vi "Get XNET Signal Names.vi"(6 "Add Info?":bool, 7 "Parent Ref in":T1 format="%.0x", 8 "error in":errorcluster, 9 "Tree In":refnum<vi>, 10 "Parent":string, 11 "Frms":refnum<k21>[](array[refnum])) -> (0 "error out":errorcluster, 1 "Tree Out":refnum<vi>, 3 "XNET Signal Names":refnum<k21>[](array[refnum]))   [LabVIEW 2015, in "Protection and Rolling Counter Addon System Explorer.lvlib"]
uses:
  Protection and Rolling Counter Addon System Explorer.lvlib
  <vilib>/NI Veristand/Custom Device API/Custom Device Item Ref.ctl
  <vilib>/NI Veristand/Custom Device API/Custom Device Channel.ctl
  <vilib>/NI Veristand/Custom Device API/Custom Device Channel Type.ctl
  Shared/SubVIs/GUID Lookup.vi
  <vilib>/NI Veristand/Custom Device API/Set Item Property (U32).vi
  <resource>/objmgr/xnet.rc
  <vilib>/NI Veristand/Custom Device API/Custom Device API.lvlib
  Shared/Protection and Rolling Counter Addon Shared.lvlib
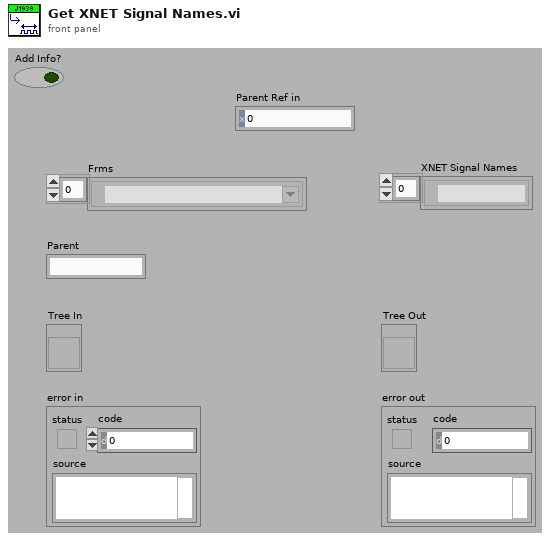
[diagram p1: front panel]
types:
  T1 = typedef "Custom Device API.lvlib/Custom Device Item Ref.ctl" = u64
  T2 = typedef "Custom Device API.lvlib/Custom Device Channel.ctl" = cluster{"Type":T3, "Units":string, "Default Value":dbl, "Faultable":bool, "Scalable":bool}
  T3 = typedef "Custom Device API.lvlib/Custom Device Channel Type.ctl" = enum16{"Input", "Output"}
  T4 = typedef "Custom Device API.lvlib/Custom Device Item Info.ctl" = cluster{"Name":string, "Is Channel":bool, "GUID":string, "Is Waveform":bool}
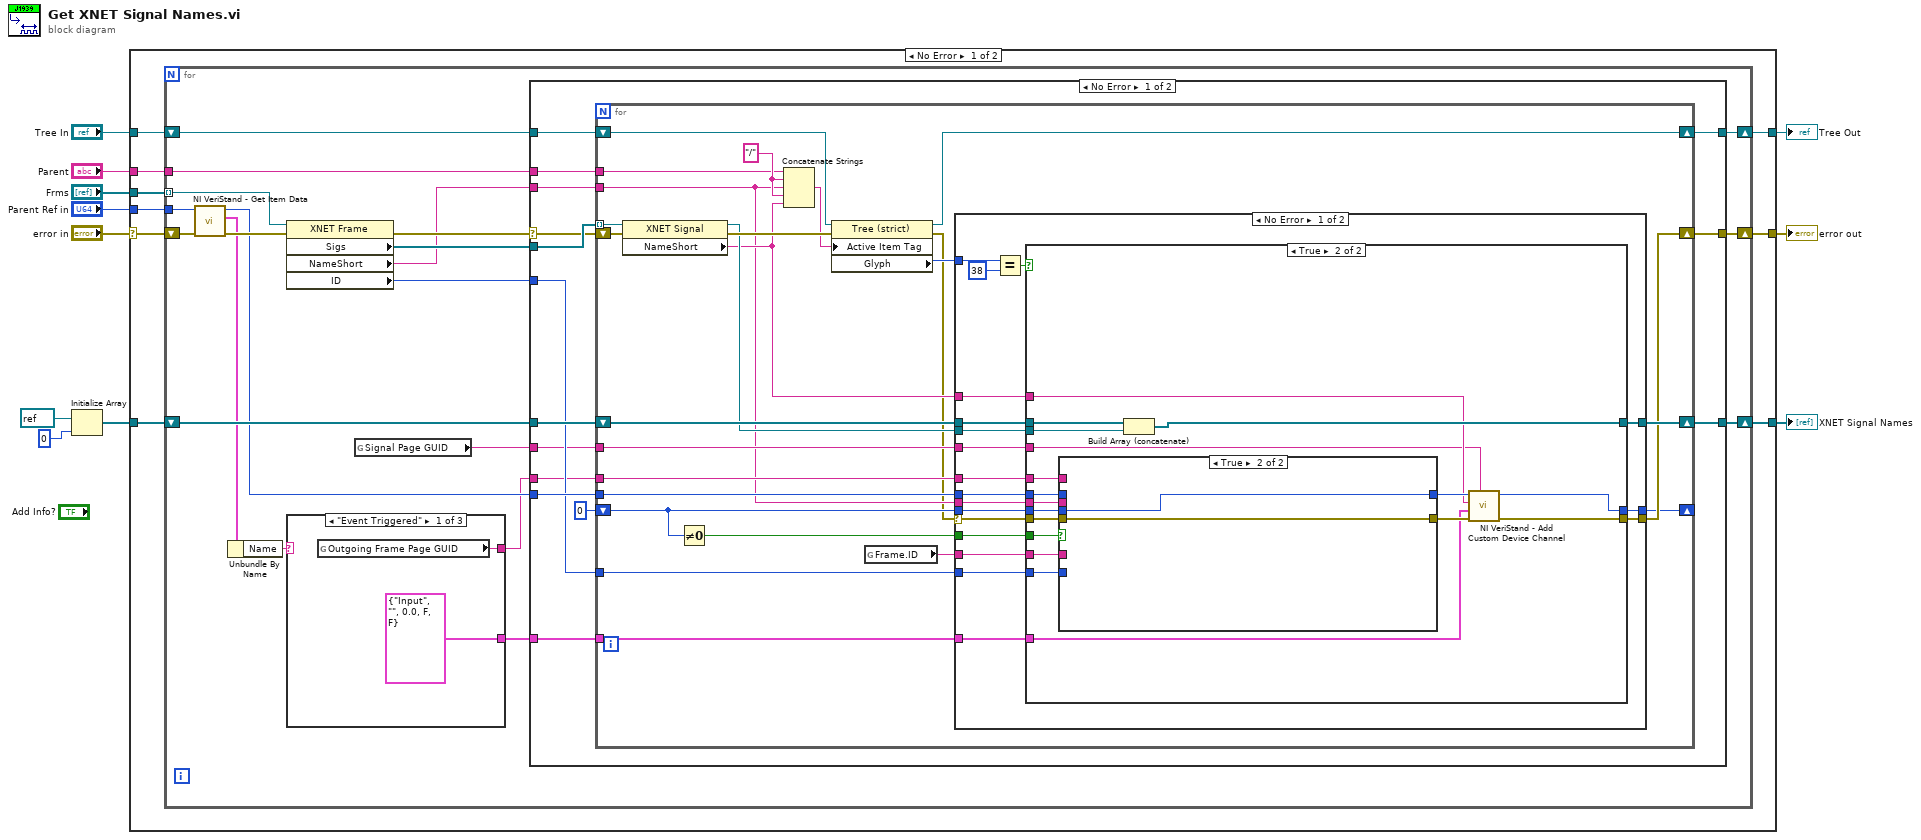
[diagram p0: block diagram]
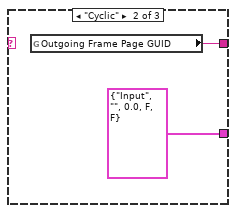
[diagram p2: hidden frame]
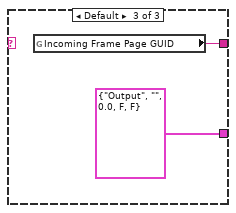
[diagram p3: hidden frame]
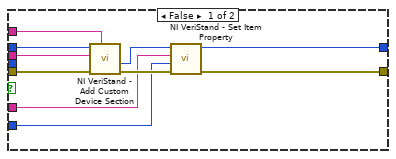
[diagram p5: hidden frame]
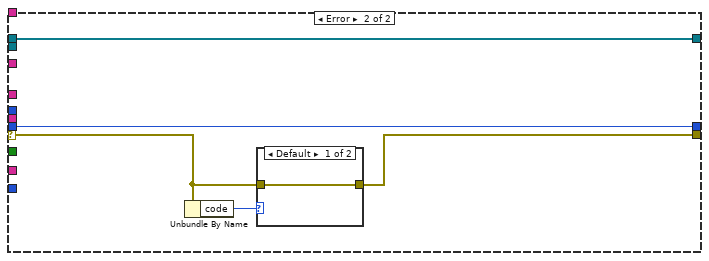
[diagram p6: hidden frame]
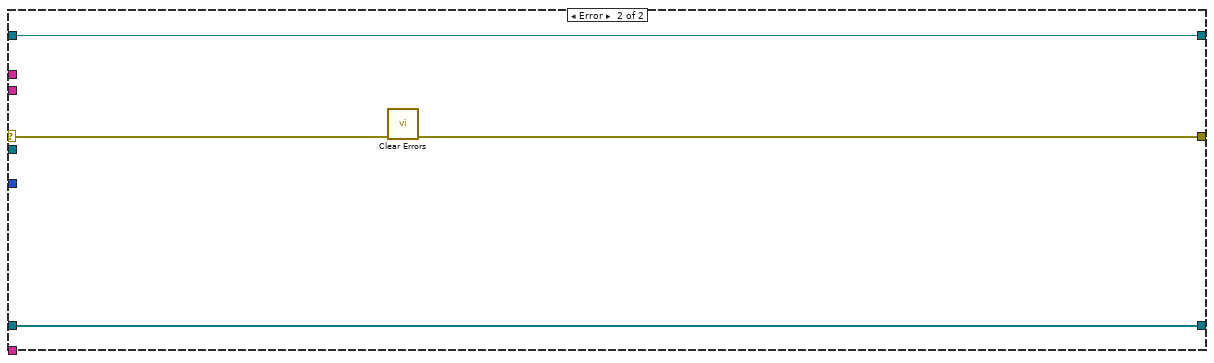
[diagram p8: hidden frame]
diagram:
  n1 = Initialize Array(refnum<k21> refnum ("XNET Signal"), 0 ("dimension size")) -> (w5:refnum<k21>[])
  n2 = case shown="No Error" "error in" {
    selector: "error in" -> [w17 w150]
    tunnel: "Parent" -> [w20 _]
    tunnel: [w19 w150] -> w10
    tunnel: "Frms" -> [w18 _]
    tunnel: [w16 _] -> w7
    tunnel: w5 -> [w15 _]
    tunnel: "Tree In" -> [w14 w149]
    tunnel: [w13 w149] -> w2
    tunnel: "Parent Ref in" -> [w12 _]
    frame No Error {
      n3 = for {
        shift-right: [w37] -> w19
        shift-left: w17 -> [w31]
        tunnel: w18 -> [w40] mode=indexing
        tunnel: w20 -> [w38]
        shift-right: [w34] -> w16
        shift-left: w15 -> [w35]
        shift-right: [w33] -> w13
        shift-left: w14 -> [w36]
        tunnel: w12 -> [w29]
        n4 = call <vilib>:"NI VeriStand - Get Item Data.vi"("error in (no error)"=w31, "Item Ref in"=w29) -> ("error out"=w30:errorcluster, "Item Info"=w27:T4, "Item Ref out"=w28:T1)  [unwired: 7 out]
        n5 = Unbundle By Name(w27) -> ("Name"=w26:string)
        n6 = property class="XNET Frame"(reference=w40, error in=w30) -> (error out=w32:errorcluster, "Sigs"=w39:refnum<k21>[], "NameShort"=w24:string, "ID"=w23:u32)  [unwired: 1 out]
        n7 = case shown="\"Event Triggered\"" w26 {
          tunnel: [T2 {"Type"=enum."Input", "Units"="", "Default Value"=0.0, "Faultable"=FALSE, "Scalable"=FALSE} ("Channel") T2 {"Type"=enum."Input", "Units"="", "Default Value"=0.0, "Faultable"=FALSE, "Scalable"=FALSE} ("Channel") T2 {"Type"=enum."Output", "Units"="", "Default Value"=0.0, "Faultable"=FALSE, "Scalable"=FALSE} ("Channel")] -> w25
          tunnel: [w41 w43 w45] -> w22
          frame "Event Triggered" {
            n8 = global read "GUID Lookup.vi" "Outgoing Frame Page GUID"() -> (w41:string)
          }
          frame "Cyclic" {
            n9 = global read "GUID Lookup.vi" "Outgoing Frame Page GUID"() -> (w43:string)
          }
          frame Default {
            n10 = global read "GUID Lookup.vi" "Incoming Frame Page GUID"() -> (w45:string)
          }
        }
        n11 = global read "GUID Lookup.vi" "Signal Page GUID"() -> (w21:string)
        n12 = case shown="No Error" w32 {
          selector: w32 -> [w51 w145]
          tunnel: w39 -> [w61 _]
          tunnel: w24 -> [w60 _]
          tunnel: w38 -> [w59 _]
          tunnel: [w58 w146] -> w37
          tunnel: w36 -> [w57 w147]
          tunnel: w35 -> [w56 w148]
          tunnel: [w55 w148] -> w34
          tunnel: [w54 w147] -> w33
          tunnel: w28 -> [w53 _]
          tunnel: w23 -> [w50 _]
          tunnel: w21 -> [w49 _]
          tunnel: w22 -> [w48 _]
          tunnel: w25 -> [w47 _]
          frame No Error {
            n13 = for {
              tunnel: w61 -> [w86] mode=indexing
              tunnel: w60 -> [w64]
              tunnel: w59 -> [w83]
              shift-right: [w74] -> w58
              shift-left: w51 -> [w85]
              shift-right: [w78] -> w55
              shift-left: w56 -> [w77]
              shift-right: [w75] -> w54
              shift-left: w57 -> [w81]
              tunnel: w53 -> [w73]
              shift-right: [w72] -> _
              shift-left: T1 0 ("Parent Ref out") -> [w71]
              tunnel: w50 -> [w68]
              tunnel: w49 -> [w67]
              tunnel: w48 -> [w66]
              tunnel: w47 -> [w65]
              w84 = "/" ("string")
              n14 = property class="XNET Signal"(reference=w86, error in=w85) -> (reference out=w76:refnum<k21>, error out=w82:errorcluster, "NameShort"=w69:string)
              n15 = Not Equal To 0?(x=w71) -> (x != 0?=w70:bool)
              n16 = Concatenate Strings(w83, w84, w64, w84, w69) -> (w80:string)
              n17 = property class="Tree (strict)"(reference=w81, error in=w82, "Active Item Tag"=w80) -> (reference out=w75:refnum<vi>, error out=w63:errorcluster, "Glyph"=w79:i32)
              n18 = global read "GUID Lookup.vi" "Frame.ID"() -> (w62:string)
              n19 = case shown="No Error" w63 {
                selector: w63 -> [w87 w140]
                tunnel: w79 -> [w105 _]
                tunnel: [w102 w142] -> w78
                tunnel: w77 -> [w101 w142]
                tunnel: w76 -> [w100 _]
                tunnel: [w99 w139] -> w74
                tunnel: w73 -> [w98 _]
                tunnel: [w97 w143] -> w72
                tunnel: w71 -> [w96 w143]
                tunnel: w70 -> [w95 _]
                tunnel: w69 -> [w94 _]
                tunnel: w68 -> [w93 _]
                tunnel: w62 -> [w92 _]
                tunnel: w67 -> [w91 _]
                tunnel: w66 -> [w90 _]
                tunnel: w65 -> [w89 _]
                tunnel: w64 -> [w88 _]
                frame No Error {
                  n20 = Equal?(x=w105, y=38) -> (x = y?=w103:bool)
                  n21 = case shown="True" w103 {
                    tunnel: [w108 w124] -> w102
                    tunnel: w101 -> [w108 w126]
                    tunnel: w100 -> [_ w125]
                    tunnel: w95 -> [_ w123]
                    tunnel: w88 -> [_ w122]
                    tunnel: w87 -> [w107 w121]
                    tunnel: [w107 w109] -> w99
                    tunnel: w98 -> [_ w120]
                    tunnel: [w106 w117] -> w97
                    tunnel: w96 -> [w106 w119]
                    tunnel: w94 -> [_ w115]
                    tunnel: w90 -> [_ w114]
                    tunnel: w91 -> [_ w113]
                    tunnel: w93 -> [_ w112]
                    tunnel: w92 -> [_ w111]
                    tunnel: w89 -> [_ w110]
                    frame False {
                    }
                    frame True {
                      n22 = case shown="True" w123 {
                        tunnel: w122 -> [w136 _]
                        tunnel: w121 -> [w135 w138]
                        tunnel: [w128 w138] -> w118
                        tunnel: w120 -> [w134 _]
                        tunnel: [w127 w137] -> w116
                        tunnel: w119 -> [_ w137]
                        tunnel: w114 -> [w133 _]
                        tunnel: w112 -> [w129 _]
                        tunnel: w111 -> [w130 _]
                        frame False {
                          n23 = call <vilib>:"NI VeriStand - Add Custom Device Section.vi"("GUID (Default Section)"=w133, "error in (no error)"=w135, "Section Name"=w136, "Parent Ref in"=w134) -> ("error out"=w131:errorcluster, "Section Ptr"=w132:T1)  [unwired: 4 in, 2 out]
                          n24 = call-poly <vilib>:"NI VeriStand - Set Item Property.vi"("error in (no error)"=w131, "Value"=w129, "Property Name"=w130, "Item Ref in"=w132) -> ("error out"=w128:errorcluster, "Item Ref out"=w127:T1)  [unwired: 5 in, 1 out]
                        }
                        frame True {
                        }
                      }
                      n25 = Build Array (concatenate)(w126, w125) -> (w124:refnum<k21>[])
                      n26 = call <vilib>:"NI VeriStand - Add Custom Device Channel.vi"("GUID (Default Channel)"=w113, "error in (no error)"=w118, "Channel"=w110, "Channel Name"=w115, "Parent Ref in"=w116) -> ("error out"=w109:errorcluster, "Parent Ref out"=w117:T1)  [unwired: 3 in, 2 out]
                    }
                  }
                }
                frame Error {
                  n27 = Unbundle By Name(w140) -> ("code"=w141:i32)
                  n28 = case shown="Default" w141 {
                    tunnel: [w144 _] -> w139
                    tunnel: w140 -> [w144 _]
                    frame Default {
                    }
                    frame 1136 {
                    }
                  }
                }
              }
            }
          }
          frame Error {
            n29 = call <vilib>:"Clear Errors.vi"("error in (no error)"=w145) -> ("error out"=w146:errorcluster)  [unwired: 5 in, 1 out]
          }
        }
      }
    }
    frame Error {
    }
  }
  "error out" <- w10
  "XNET Signal Names" <- w7
  "Tree Out" <- w2
